vi "1010.vi"() -> ()   [LabVIEW 2015]
uses:
  <vilib>/NXT/Block Support/NXT_InputPort.ctl
  <vilib>/NXT/Block Support/NXT_OutputPort.ctl
  <vilib>/NXT/Dual Mode Library/Sensors/Sonar_cm.vi
  <vilib>/NXT/NXTIO Xnodes/NXTIONodeSubVIs/NXTMoveMotors.vi
  <vilib>/NXT/Dual Mode Library/Sensors/Light_On.vi
  <vilib>/NXT/NXTIO Xnodes/NXTIONodeSubVIs/LEGOStopAllMotors.vi
  <vilib>/NXT/Dual Mode Library/Waits/Wait_Num.vi
  <vilib>/NXT/Subs/LVHSConnector.ctl
  <vilib>/NXT/NXTIO Xnodes/AddressXNode/NXTIOAddress.xnode
  <vilib>/NXT/NXTIO Xnodes/NXTIOXNode/NXTIO.xnode
  <vilib>/NXT/LegoClasses/BrickReference/BrickReference.lvclass
panel:
  in  "stop":bool
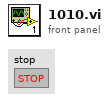
[diagram p1: front panel]
types:
  T1 = typedef "NXT_OutputPort.ctl" = u8
  T2 = typedef "NXT_InputPort.ctl" = u32
  T3 = typedef "LVHSConnector.ctl" = refnum<class "BrickReference.lvclass">
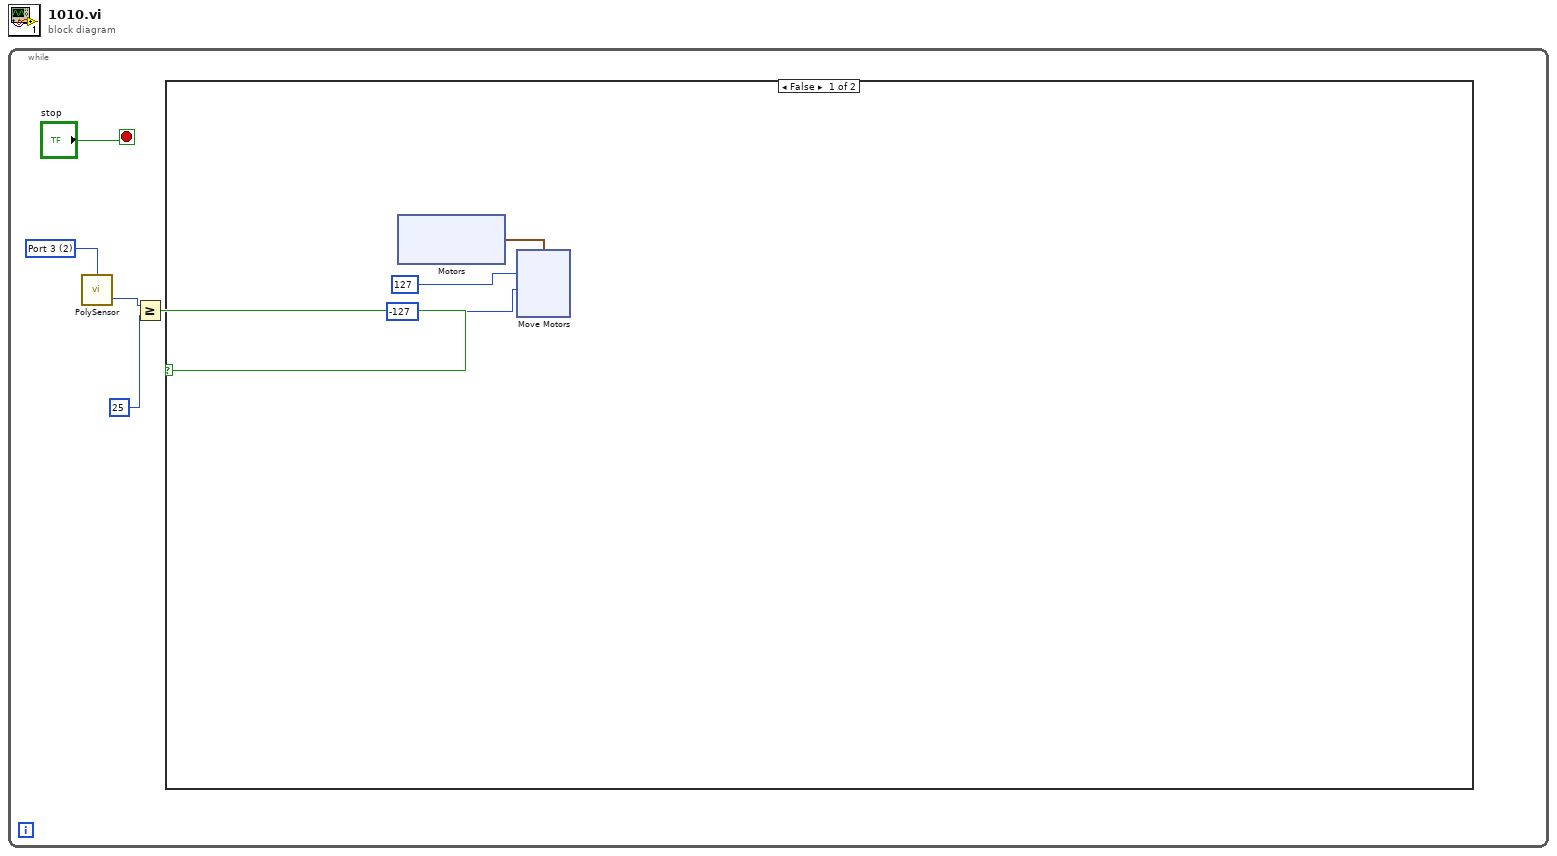
[diagram p0: block diagram]
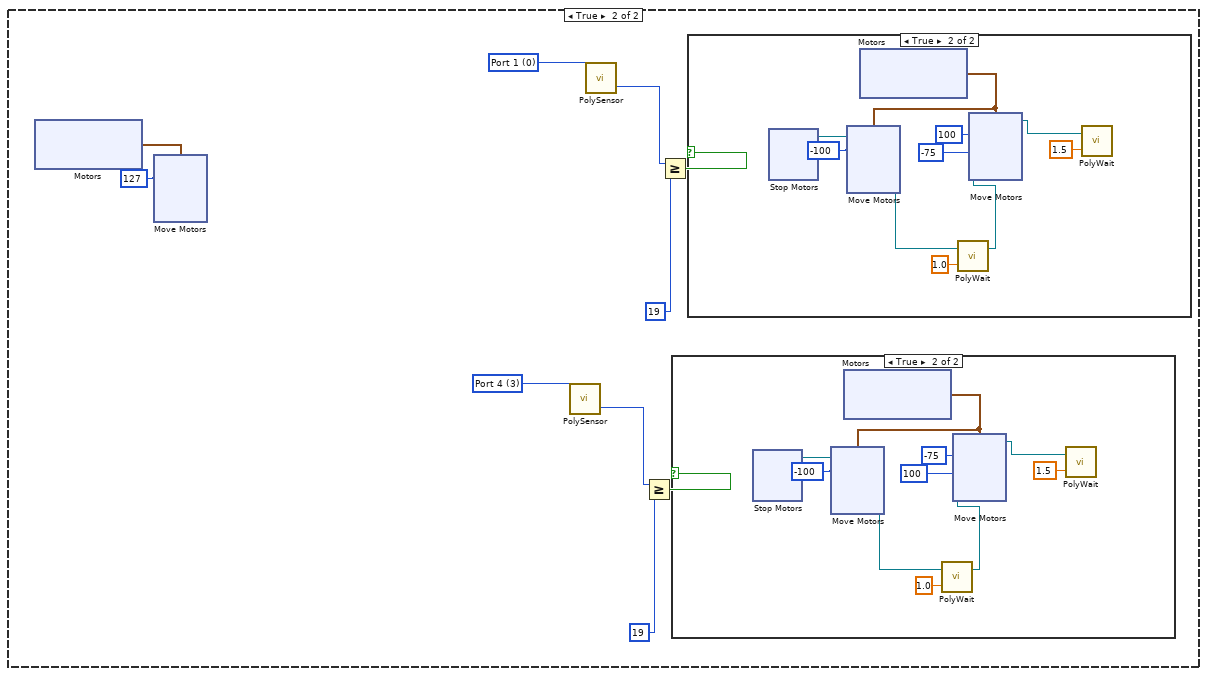
[diagram p2: hidden frame]
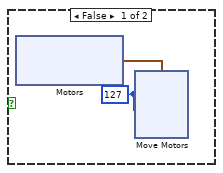
[diagram p3: hidden frame]
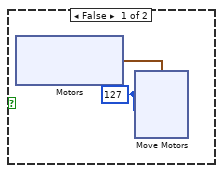
[diagram p4: hidden frame]
diagram:
  n1 = while {
    stop <- "stop" stop-if-true
    w5 = T2 2 items=["Port 1", "Port 2", "Port 3", "Port 4"] ("Port (Port 4)")
    n2 = call-poly <vilib>:"PolySensor.vi"("Port (Port 4)"=w5) -> ("Distance (cm)"=w4:i16)  [unwired: 2 in, 1 out]
    n3 = Greater Or Equal?(x=w4, y=i16 25) -> (x >= y?=w2:bool)
    n4 = case shown="False" w2 {
      frame False {
        n5 = xnode "Motors"() -> ("Motor"=w8:cluster{"Port":T1, "Port":T1})
        n6 = xnode "Move Motors"("Power/Speed 2"=i8 -127, "Power/Speed 1"=i8 127, "Motors"=w8) -> ()  [unwired: 1 in, 1 out]
      }
      frame True {
        w18 = T2 3 items=["Port 1", "Port 2", "Port 3", "Port 4"] ("Port (Port 3)")
        w22 = i8 127 ("Power/Speed 1")
        w24 = T2 0 items=["Port 1", "Port 2", "Port 3", "Port 4"] ("Port (Port 3)")
        n7 = xnode "Motors"() -> ("Motor"=w23:cluster{"Port":T1, "Port":T1})
        n8 = xnode "Move Motors"("Power/Speed 1"=w22, "Motors"=w23, "Power/Speed 2"=w22) -> ()  [unwired: 1 in, 1 out]
        n9 = call-poly <vilib>:"PolySensor.vi"("Port (Port 3)"=w18) -> ("Scaled Value"=w20:i16)  [unwired: 2 in, 1 out]
        n10 = call-poly <vilib>:"PolySensor.vi"("Port (Port 3)"=w24) -> ("Scaled Value"=w26:i16)  [unwired: 2 in, 1 out]
        n11 = Greater Or Equal?(x=w20, y=i16 19) -> (x >= y?=w21:bool)
        n12 = Greater Or Equal?(x=w26, y=i16 19) -> (x >= y?=w27:bool)
        n13 = case shown="True" w21 {
          frame False {
            w28 = i8 127 ("Power/Speed 1")
            n14 = xnode "Motors"() -> ("Motor"=w29:cluster{"Port":T1, "Port":T1})
            n15 = xnode "Move Motors"("Power/Speed 2"=w28, "Power/Speed 1"=w28, "Motors"=w29) -> ()  [unwired: 1 in, 1 out]
          }
          frame True {
            w43 = i8 -100 ("Power/Speed 1")
            n16 = xnode "Stop Motors"() -> ("NXT/EV3"=w39:T3)  [unwired: 2 in]
            n17 = xnode "Motors"() -> ("Motor"=w44:cluster{"Port":T1, "Port":T1})
            n18 = xnode "Move Motors"("Power/Speed 2"=w43, "Power/Speed 1"=w43, "Motors"=w44, "NXT/EV3"=w39) -> ("NXT/EV3"=w42:T3)
            n19 = call-poly <vilib>:"PolyWait.vi"("Time (1 sec)"=sgl 1.0, "NXT/EV3"=w42) -> ("NXT/EV3"=w41:T3)  [unwired: 2 in]
            n20 = xnode "Move Motors"("Power/Speed 2"=i8 100, "Power/Speed 1"=i8 -75, "Motors"=w44, "NXT/EV3"=w41) -> ("NXT/EV3"=w48:T3)
            n21 = call-poly <vilib>:"PolyWait.vi"("Time (1 sec)"=sgl 1.5, "NXT/EV3"=w48) -> ()  [unwired: 2 in, 1 out]
          }
        }
        n22 = case shown="True" w27 {
          frame False {
            w78 = i8 127 ("Power/Speed 1")
            n23 = xnode "Motors"() -> ("Motor"=w79:cluster{"Port":T1, "Port":T1})
            n24 = xnode "Move Motors"("Power/Speed 2"=w78, "Power/Speed 1"=w78, "Motors"=w79) -> ()  [unwired: 1 in, 1 out]
          }
          frame True {
            w93 = i8 -100 ("Power/Speed 1")
            n25 = xnode "Stop Motors"() -> ("NXT/EV3"=w89:T3)  [unwired: 2 in]
            n26 = xnode "Motors"() -> ("Motor"=w94:cluster{"Port":T1, "Port":T1})
            n27 = xnode "Move Motors"("Power/Speed 2"=w93, "Power/Speed 1"=w93, "Motors"=w94, "NXT/EV3"=w89) -> ("NXT/EV3"=w92:T3)
            n28 = call-poly <vilib>:"PolyWait.vi"("Time (1 sec)"=sgl 1.0, "NXT/EV3"=w92) -> ("NXT/EV3"=w91:T3)  [unwired: 2 in]
            n29 = xnode "Move Motors"("Power/Speed 2"=i8 -75, "Power/Speed 1"=i8 100, "Motors"=w94, "NXT/EV3"=w91) -> ("NXT/EV3"=w98:T3)
            n30 = call-poly <vilib>:"PolyWait.vi"("Time (1 sec)"=sgl 1.5, "NXT/EV3"=w98) -> ()  [unwired: 2 in, 1 out]
          }
        }
      }
    }
  }
